vi "get Tx Rx Result.vi"(8 "error in (no error)":errorcluster, 10 "result":i32, 11 "protocol_version":i32) -> (0 "error out":errorcluster, 3 "function return":string)   [LabVIEW 2018, in "labview.lvlib"]
doc: "WINDECLSPEC const char *getTxRxResult (int protocol_version, int result);"
uses:
  labview.lvlib
  dxl_x86_c.dll
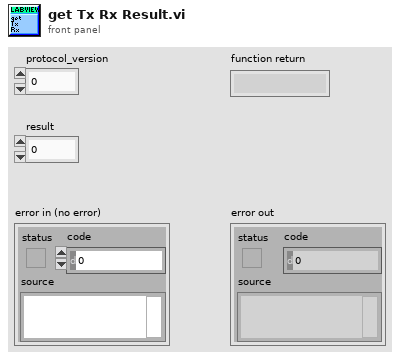
[diagram p1: front panel]
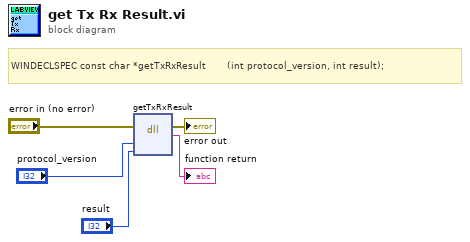
[diagram p0: block diagram]
diagram:
  # "WINDECLSPEC const char *getTxRxResult       (int protocol_version, int result);"
  n1 = dll-call lib="C:/Users/joaos/OneDrive/Documents/[PhD]/Project Omnidirectional Vehicle/Vanes/LabView_code/joaoandthethreestands/DynamixelSDK-3.7.31/labview/new_compilation/dxl_x86_c.*" fn="getTxRxResult"(error in="error in (no error)", "protocol_version"="protocol_version", "result"="result") -> (error out=→"error out":errorcluster, →"function return":string)  [unwired: 4 in, 1 out]
